vi "PAQmem_destructor.vi"(8 "error in (no error)":errorcluster, 11 "PAQ-memory in":refnum<class "PAQ-memory.lvclass">) -> (0 "error out":errorcluster, 3 "PAQ-memory out":refnum<class "PAQ-memory.lvclass">)   [LabVIEW 2014, in "PAQ-memory.lvclass"]
doc: "Close all references within this object"
uses:
  PAQ-memory.lvclass
  PAQ-memory.lvclass/PAQ-memory.ctl
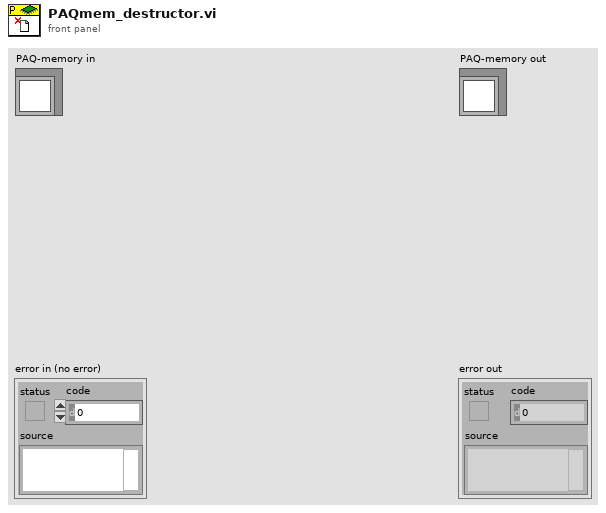
[diagram p1: front panel]
types:
  T1 = cluster{"source":refnum<data-value>, "status":refnum<data-value>, "data":refnum<data-value>, "max":refnum<data-value>, "min":refnum<data-value>}[]
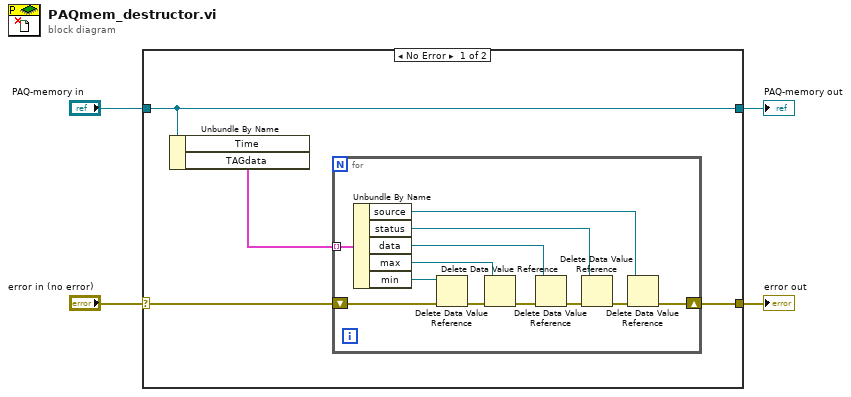
[diagram p0: block diagram]
diagram:
  n1 = case shown="No Error" "error in (no error)" {
    selector: "error in (no error)" -> [w6 w22]
    tunnel: [w5 w22] -> w3
    tunnel: [w8 w21] -> w1
    tunnel: "PAQ-memory in" -> [w8 w21]
    frame No Error {
      n2 = Unbundle By Name(w8) -> ("TAGdata"=w7:T1)  [unwired: 1 out]
      n3 = for {
        tunnel: w7 -> [w20] mode=indexing
        shift-right: [w9] -> w5
        shift-left: w6 -> [w14]
        n4 = Unbundle By Name(w20) -> ("source"=w15:refnum<data-value>, "status"=w16:refnum<data-value>, "data"=w17:refnum<data-value>, "max"=w18:refnum<data-value>, "min"=w19:refnum<data-value>)
        n5 = Delete Data Value Reference(data value reference=w19, error in=w14) -> (error out=w13:errorcluster)  [unwired: 1 out]
        n6 = Delete Data Value Reference(data value reference=w18, error in=w13) -> (error out=w12:errorcluster)  [unwired: 1 out]
        n7 = Delete Data Value Reference(data value reference=w17, error in=w12) -> (error out=w11:errorcluster)  [unwired: 1 out]
        n8 = Delete Data Value Reference(data value reference=w16, error in=w11) -> (error out=w10:errorcluster)  [unwired: 1 out]
        n9 = Delete Data Value Reference(data value reference=w15, error in=w10) -> (error out=w9:errorcluster)  [unwired: 1 out]
      }
    }
    frame Error {
    }
  }
  "error out" <- w3
  "PAQ-memory out" <- w1
